vi "load_class.vi"   [LabVIEW 2015, in "lv-post-installer.lvlib"]
uses:
  lv-post-installer.lvlib
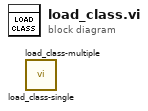
[diagram p0: block diagram]
diagram:
  n1 = call "load_class-single.vi"() -> ()  [unwired: 10 in, 2 out]
  n2 = call "load_class-multiple.vi"() -> ()  [unwired: 10 in, 2 out]
